vi "Create Target Folders.vi"(8 "error in (no error)":errorcluster, 10 "Target Names in":string[](array[string]), 11 "Project Sync Tools in":refnum<class "Project Sync Tools.lvclass">) -> (0 "error out":errorcluster, 2 "RT Targets Folders":path[](array[path]), 3 "Project Sync Tools out":refnum<class "Project Sync Tools.lvclass">)   [LabVIEW 2019, in "Project Sync Tools.lvclass"]
uses:
  Project Sync Tools.lvclass
  Project Sync Tools.lvclass/Project Sync Tools.ctl
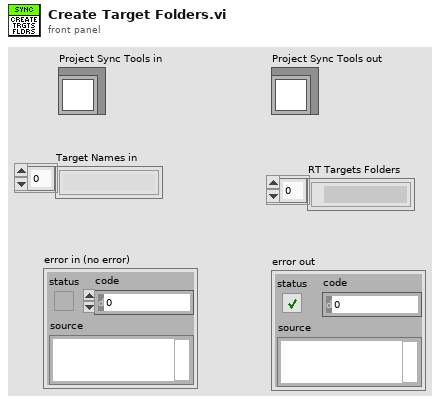
[diagram p1: front panel]
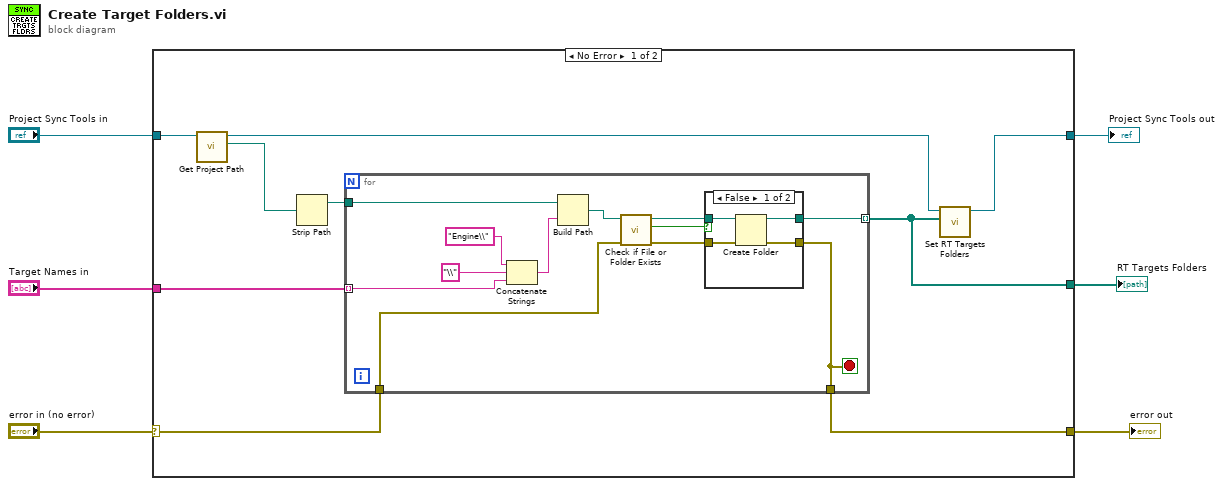
[diagram p0: block diagram]
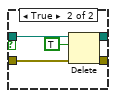
[diagram p2: hidden frame]
diagram:
  n1 = case shown="No Error" "error in (no error)" {
    selector: "error in (no error)" -> [w8 w38]
    tunnel: [w15 w37] -> w6
    tunnel: "Project Sync Tools in" -> [w12 w37]
    tunnel: [w10 w38] -> w3
    tunnel: [w9 _] -> w2
    tunnel: "Target Names in" -> [w7 _]
    frame No Error {
      n2 = call "Get Project Path.vi"("CD Build Tools in"=w12) -> ("Project Path"=w11:path, "CD Build Tools out"=w14:refnum<class "Project Sync Tools.lvclass">)  [unwired: 9 in]
      n3 = Strip Path(path=w11) -> (stripped path=w13:path)  [unwired: 1 out]
      n4 = for {
        tunnel: w13 -> [w20]
        tunnel: [w19] -> w9 mode=indexing
        tunnel: [w18] -> w10
        tunnel: w8 -> [w16]
        tunnel: w7 -> [w17] mode=indexing
        stop <- w18 stop-if-true
        n5 = Concatenate Strings("Engine\\" ("name or relative path"), "\\" ("string"), w17) -> (w26:string)
        n6 = Build Path(base path=w20, name or relative path=w26) -> (appended path=w25:path)
        n7 = call <vilib>:"Check if File or Folder Exists.vi"("error in (no error)"=w16, "path"=w25) -> ("error out"=w22:errorcluster, "file or folder exists?"=w24:bool, "dup path"=w23:path)  [unwired: 7 in]
        n8 = case shown="False" w24 {
          tunnel: w23 -> [w31 w36]
          tunnel: w22 -> [w30 w34]
          tunnel: [w29 w33] -> w19
          tunnel: [w28 w32] -> w18
          frame False {
            n9 = Create Folder(path (use dialog)=w31, error in=w30) -> (created path=w29:path, error out=w28:errorcluster)  [unwired: 1 in, 1 out]
          }
          frame True {
            n10 = Delete(path (use dialog)=w36, entire hierarchy (F)=TRUE, error in=w34) -> (deleted path=w33:path, error out=w32:errorcluster)  [unwired: 2 in, 1 out]
          }
        }
      }
      n11 = call "Set RT Targets Folders.vi"("RT Targets Folders"=w9, "Project Sync Tools in"=w14) -> ("Project Sync Tools out"=w15:refnum<class "Project Sync Tools.lvclass">)  [unwired: 9 in]
    }
    frame Error {
    }
  }
  "Project Sync Tools out" <- w6
  "error out" <- w3
  "RT Targets Folders" <- w2
